vi "WriteIniFiles_ByVarient.vi"(8 "error in (no error)":errorcluster, 10 "Variant":variant, 11 "path":path) -> (0 "error out":errorcluster)   [LabVIEW 2017]
uses:
  <vilib>/Utility/config.llb/NI_LVConfig.lvlib
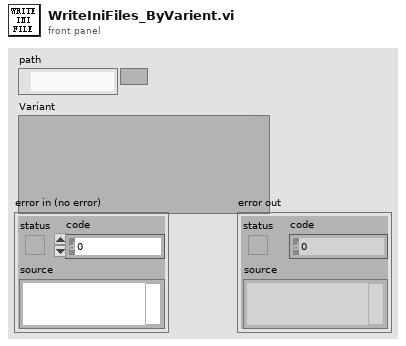
[diagram p1: front panel]
types:
  T1 = typedef "NI_LVConfig.lvlib/Config Data RefNum.ctl" = refnum<k1>
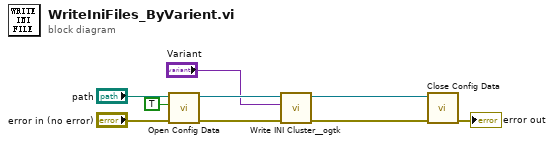
[diagram p0: block diagram]
diagram:
  n1 = call <vilib>:"Open Config Data.vi"("error in (no error)"="error in (no error)", "create file if necessary (T)"=TRUE, "configuration file path"="path") -> ("error out"=w3:errorcluster, "refnum"=w5:T1)  [unwired: 6 in, 1 out]
  n2 = call "Write INI Cluster__ogtk.vi"("error in (no error)"=w3, "INI Fomatted Cluster"="Variant", "refnum"=w5) -> ("error out"=w1:errorcluster, "dup refnum"=w4:T1)  [unwired: 7 in]
  n3 = call <vilib>:"Close Config Data.vi"("error in (no error)"=w1, "refnum"=w4) -> ("error out"=→"error out":errorcluster)  [unwired: 8 in, 1 out]
